vi "假的lumitrax.vi"() -> ()   [LabVIEW 2015]
uses:
  <vilib>/vision/NI_Vision_Development_Module.lvlib
panel:
  out "Image 2":T1(plugin-control)
  out "Image":T1(plugin-control)
  out "x-y":dbl
  out "Left":T1(plugin-control)
  out "Up":T1(plugin-control)
  out "Right":T1(plugin-control)
  out "Down":T1(plugin-control)
  out "Array":T1[][](array[plugin-control])
  out "UD":T1(plugin-control)
  out "Ave":T1(plugin-control)
  out "UDLR":T1(plugin-control)
  out "LR":T1(plugin-control)
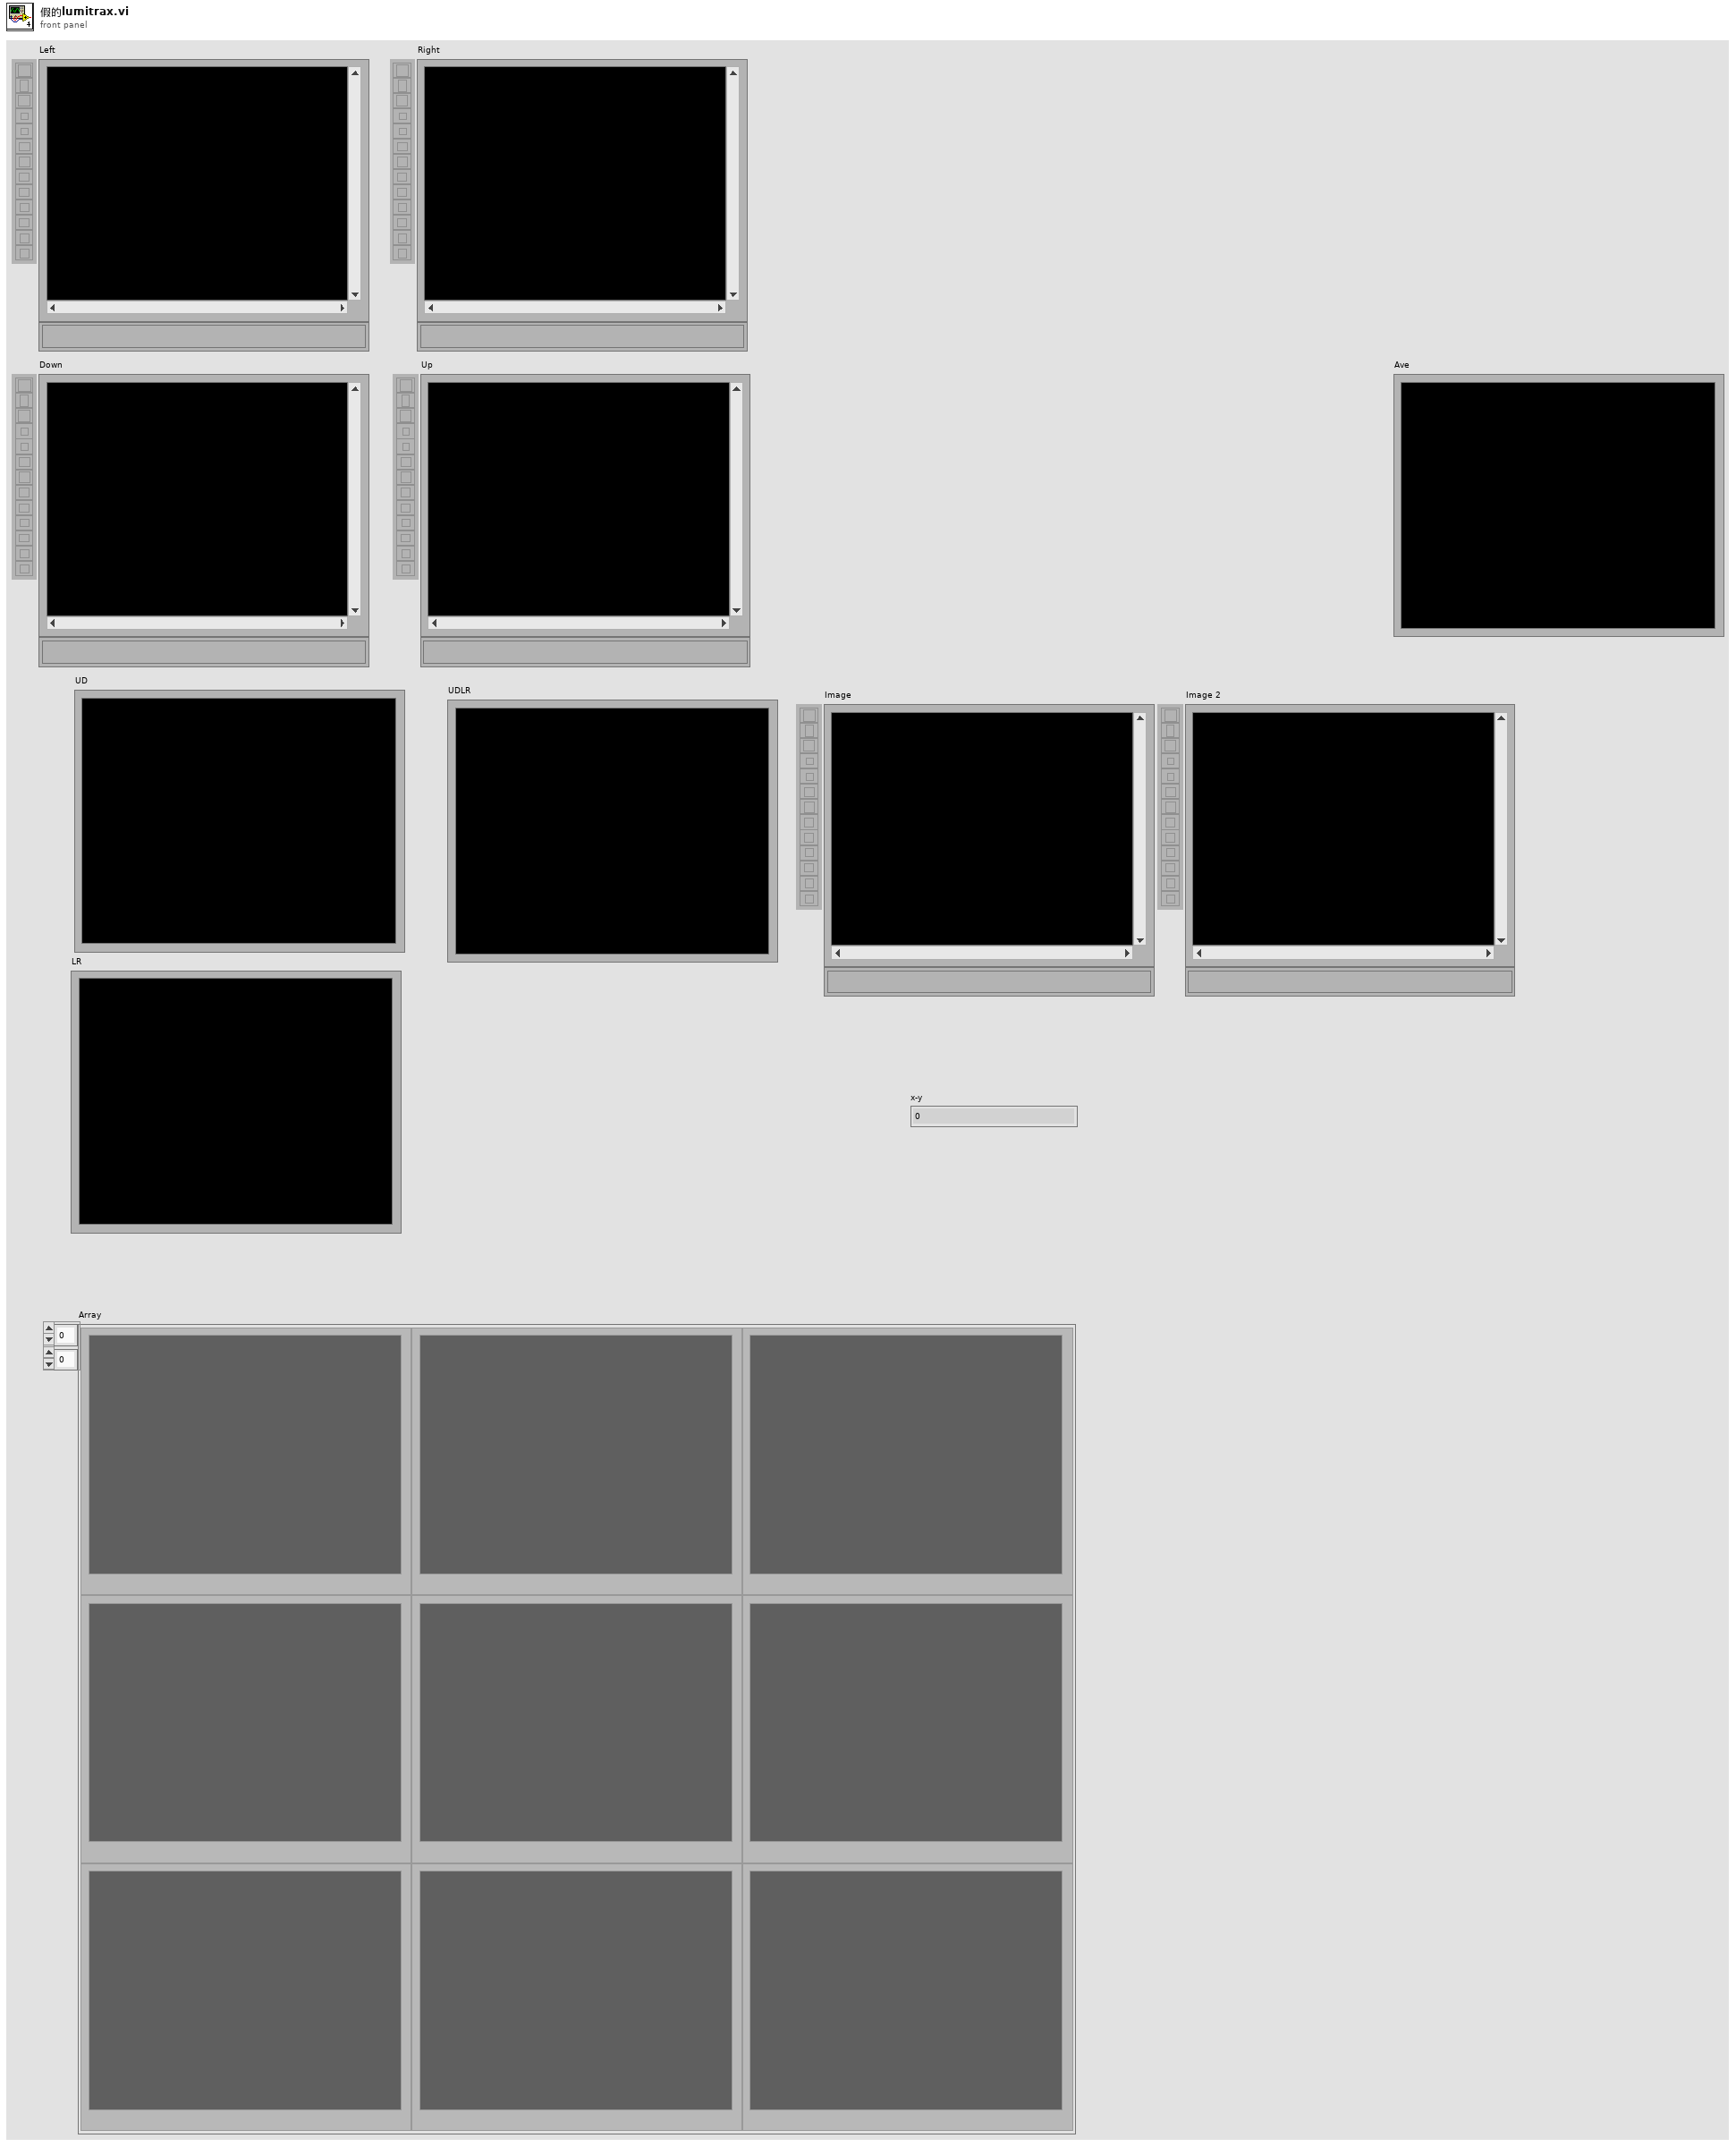
[diagram p1: front panel]
types:
  T1 = typedef "IMAQ Image.ctl" = refnum<image>
  T2 = cluster{"Line Scan Image?":bool, "Correction Factor":sgl}
  T3 = cluster{"Model":i32, "Sampling Grid Size":cluster{"SizeX":i32, "SizeY":i32}, "Polynomial Degree":i32}
  T4 = cluster{"Estimate Background?":bool, "Method":i32, "Polynomial Degree":i32, "Window Size (32x32)":cluster{"SizeX":i32, "SizeY":i32}, "Niblack Deviation Factor (0.2)":dbl}
  T5 = typedef "Image Type" = u32
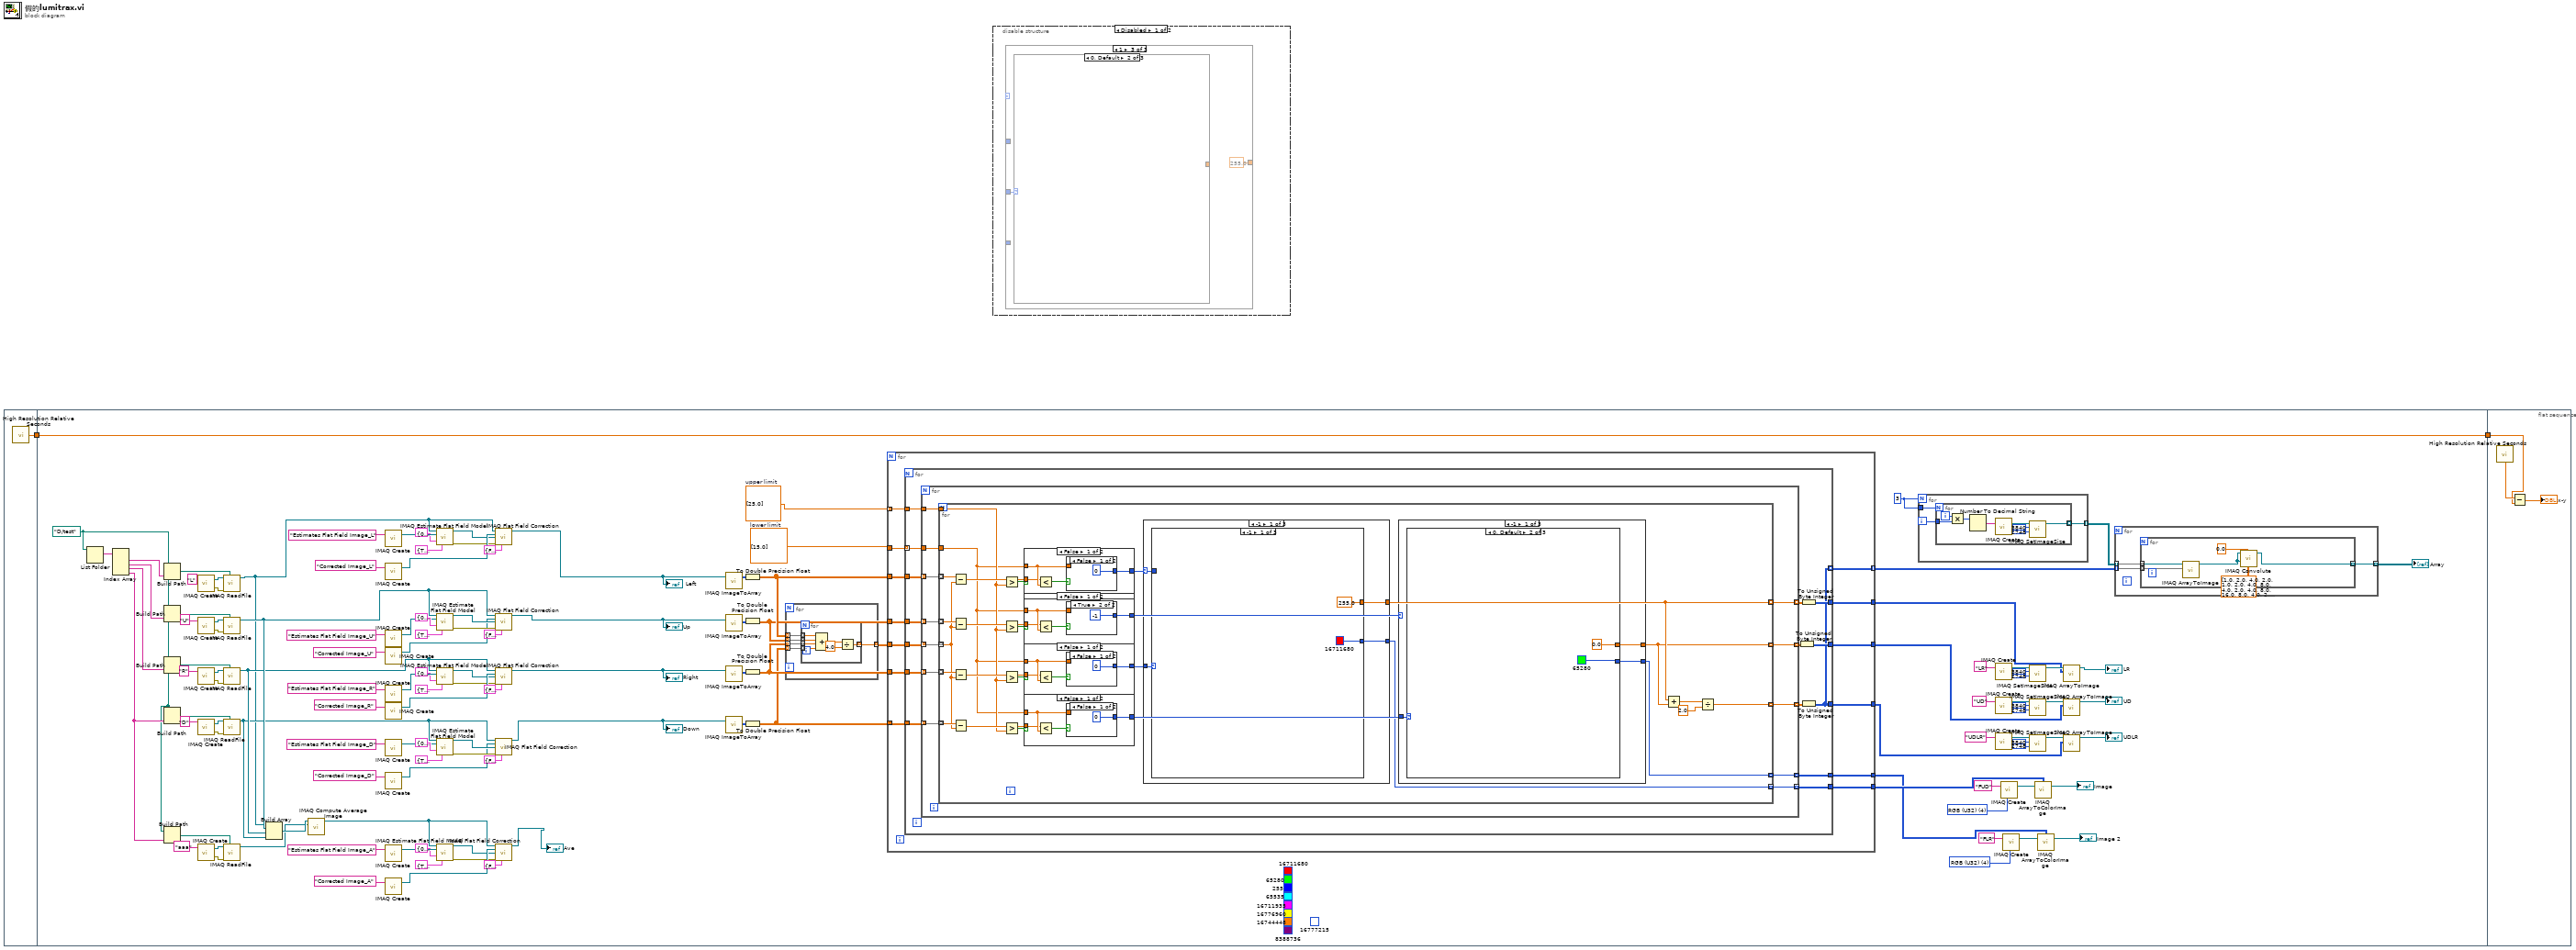
[diagram p0: block diagram]
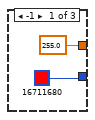
[diagram p2: hidden frame]
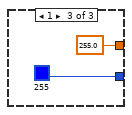
[diagram p3: hidden frame]
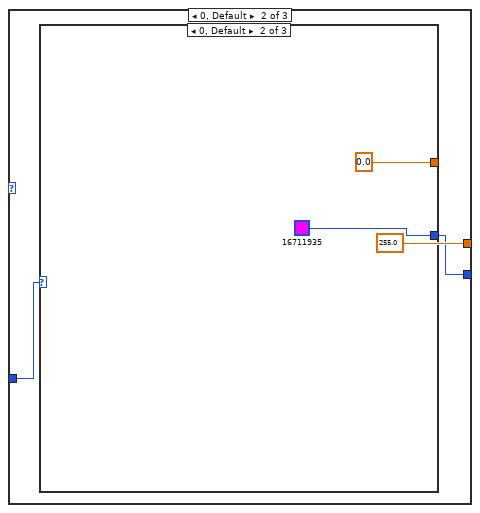
[diagram p4: hidden frame]
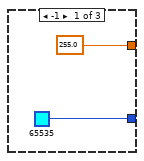
[diagram p5: hidden frame]
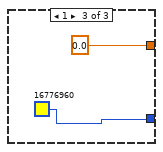
[diagram p6: hidden frame]
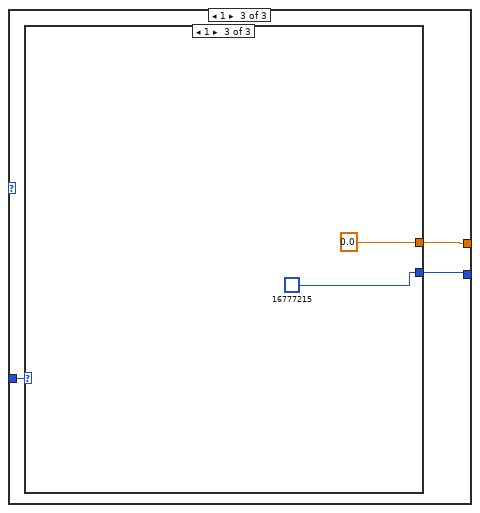
[diagram p7: hidden frame]
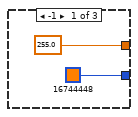
[diagram p8: hidden frame]
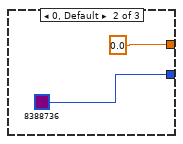
[diagram p9: hidden frame]
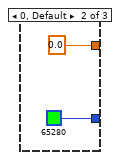
[diagram p10: hidden frame]
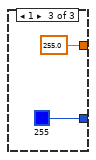
[diagram p11: hidden frame]
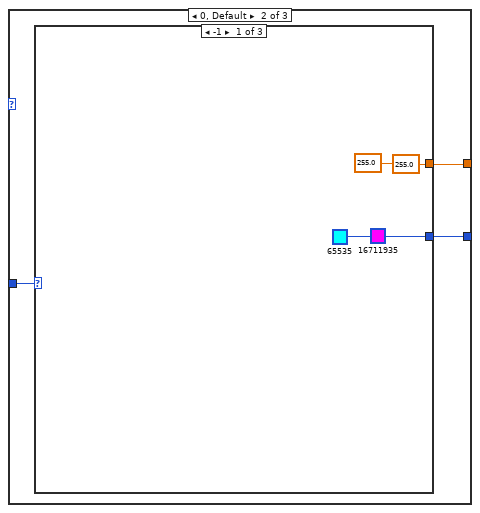
[diagram p12: hidden frame]
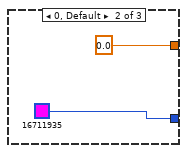
[diagram p13: hidden frame]
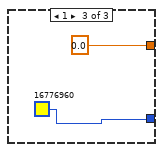
[diagram p14: hidden frame]
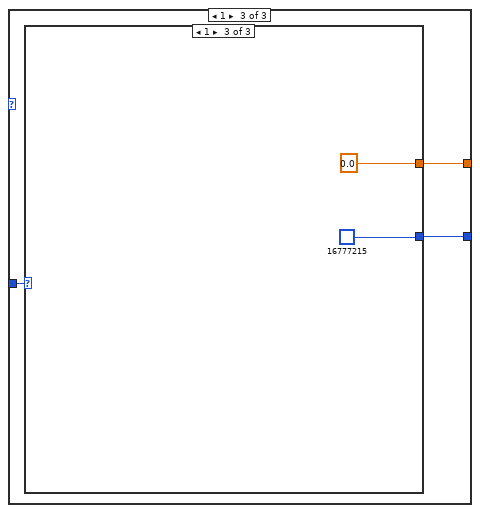
[diagram p15: hidden frame]
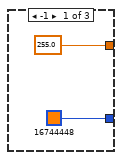
[diagram p16: hidden frame]
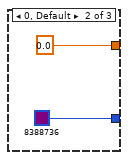
[diagram p17: hidden frame]
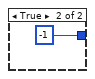
[diagram p18: hidden frame]
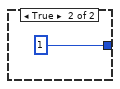
[diagram p19: hidden frame]
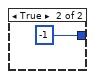
[diagram p20: hidden frame]
diagram:
  n1 = flat-sequence {
    tunnel: [w3] -> w2
    tunnel: w2 -> [w16]
    tunnel: [w16] -> w1
    tunnel: w1 -> [w316]
    frame #0 {
      n2 = call <vilib>:"High Resolution Relative Seconds.vi"() -> ("relative seconds"=w3:dbl)
    }
    frame #1 {
      w8 = T5 4 items=["Grayscale (U8)", "Grayscale (I16)", "Grayscale (SGL)", "Complex (CSG)", "RGB (U32)", "HSL (U32)", "RGB (U64)", "Grayscale (U16)"] ("Image Type")
      w9 = T5 4 items=["Grayscale (U8)", "Grayscale (I16)", "Grayscale (SGL)", "Complex (CSG)", "RGB (U32)", "HSL (U32)", "RGB (U64)", "Grayscale (U16)"] ("Image Type")
      (unwired) u32 16777215 ("O")
      (unwired) u32 8388736 ("P")
      (unwired) u32 16744448 ("O")
      (unwired) u32 16776960 ("Y")
      (unwired) u32 65535 ("C")
      (unwired) u32 16711935 ("M")
      (unwired) u32 255 ("B")
      (unwired) u32 65280 ("G")
      (unwired) u32 16711680 ("R")
      w14 = dbl[] [15.0]  # lower limit
      w15 = dbl[] [25.0]  # upper limit
      w26 = path "D:/test"
      w121 = 3
      n3 = List Folder(path=w26) -> (filenames=w119:string[])  [unwired: 3 in, 3 out]
      n4 = Index Array(array=w119) -> (element #1=w118:string, element #2=w116:string, element #3=w117:string, element #4=w43:string)  [unwired: 4 in]
      n5 = Build Path(base path=w26, name or relative path=w118) -> (appended path=w115:path)
      n6 = Build Path(base path=w26, name or relative path=w116) -> (appended path=w114:path)
      n7 = Build Path(base path=w26, name or relative path=w117) -> (appended path=w113:path)
      n8 = Build Path(base path=w26, name or relative path=w43) -> (appended path=w112:path)
      n9 = Build Path(base path=w26, name or relative path=w43) -> (appended path=w47:path)
      n10 = call "IMAQ Create"("Image Name"="L") -> ("New Image"=w128:T1, "error out"=w129:errorcluster)  [unwired: 4 in]
      n11 = call "IMAQ Create"("Image Name"="U") -> ("New Image"=w126:T1, "error out"=w127:errorcluster)  [unwired: 4 in]
      n12 = call "IMAQ Create"("Image Name"="R") -> ("New Image"=w124:T1, "error out"=w125:errorcluster)  [unwired: 4 in]
      n13 = call "IMAQ Create"("Image Name"="D") -> ("New Image"=w122:T1, "error out"=w123:errorcluster)  [unwired: 4 in]
      n14 = call "IMAQ Create"("Image Name"="aaa") -> ("New Image"=w46:T1, "error out"=w45:errorcluster)  [unwired: 4 in]
      n15 = call "IMAQ ReadFile"("File Path"=w115, "error in (no error)"=w129, "Image"=w128) -> ("Image Out"=w27:T1)  [unwired: 4 in, 4 out]
      n16 = call "IMAQ ReadFile"("File Path"=w114, "error in (no error)"=w127, "Image"=w126) -> ("Image Out"=w42:T1)  [unwired: 4 in, 4 out]
      n17 = call "IMAQ ReadFile"("File Path"=w113, "error in (no error)"=w125, "Image"=w124) -> ("Image Out"=w41:T1)  [unwired: 4 in, 4 out]
      n18 = call "IMAQ ReadFile"("File Path"=w112, "error in (no error)"=w123, "Image"=w122) -> ("Image Out"=w40:T1)  [unwired: 4 in, 4 out]
      n19 = call "IMAQ ReadFile"("File Path"=w47, "error in (no error)"=w45, "Image"=w46) -> ("Image Out"=w38:T1)  [unwired: 4 in, 4 out]
      n20 = Build Array(w27, w42, w41, w40) -> (w39:T1[])
      n21 = call "IMAQ Compute Average Image"("Image Dst"=w38, "Images"=w39) -> ("Image Dst Out"=w28:T1)  [unwired: 8 in, 1 out]
      n22 = call "IMAQ Create"("Image Name"="Estimates Flat Field Image_L") -> ("New Image"=w84:T1)  [unwired: 4 in, 1 out]
      n23 = call "IMAQ Create"("Image Name"="Corrected Image_L") -> ("New Image"=w85:T1)  [unwired: 4 in, 1 out]
      n24 = call "IMAQ Create"("Image Name"="Estimates Flat Field Image_U") -> ("New Image"=w73:T1)  [unwired: 4 in, 1 out]
      n25 = call "IMAQ Create"("Image Name"="Corrected Image_U") -> ("New Image"=w72:T1)  [unwired: 4 in, 1 out]
      n26 = call "IMAQ Create"("Image Name"="Estimates Flat Field Image_R") -> ("New Image"=w66:T1)  [unwired: 4 in, 1 out]
      n27 = call "IMAQ Create"("Image Name"="Corrected Image_R") -> ("New Image"=w67:T1)  [unwired: 4 in, 1 out]
      n28 = call "IMAQ Create"("Image Name"="Estimates Flat Field Image_D") -> ("New Image"=w55:T1)  [unwired: 4 in, 1 out]
      n29 = call "IMAQ Create"("Image Name"="Corrected Image_D") -> ("New Image"=w54:T1)  [unwired: 4 in, 1 out]
      n30 = call "IMAQ Create"("Image Name"="Estimates Flat Field Image_A") -> ("New Image"=w35:T1)  [unwired: 4 in, 1 out]
      n31 = call "IMAQ Create"("Image Name"="Corrected Image_A") -> ("New Image"=w36:T1)  [unwired: 4 in, 1 out]
      n32 = call "IMAQ Estimate Flat Field Model"("Image Src"=w27, "Image Dst"=w84, "Surface Fit Options"=T3 {"Model"=0, "Sampling Grid Size"={"SizeX"=100, "SizeY"=100}, "Polynomial Degree"=3}, "Background Estimation Options"=T4 {"Estimate Background?"=TRUE, "Method"=0, "Polynomial Degree"=2, "Window Size (32x32)"={"SizeX"=32, "SizeY"=32}, "Niblack Deviation Factor (0.2)"=0.2}) -> ("Flat Field Image Out"=w83:T1, "error out"=w81:errorcluster)  [unwired: 10 in]
      n33 = call "IMAQ Estimate Flat Field Model"("Image Src"=w42, "Image Dst"=w73, "Surface Fit Options"=T3 {"Model"=0, "Sampling Grid Size"={"SizeX"=100, "SizeY"=100}, "Polynomial Degree"=3}, "Background Estimation Options"=T4 {"Estimate Background?"=TRUE, "Method"=0, "Polynomial Degree"=2, "Window Size (32x32)"={"SizeX"=32, "SizeY"=32}, "Niblack Deviation Factor (0.2)"=0.2}) -> ("Flat Field Image Out"=w74:T1, "error out"=w76:errorcluster)  [unwired: 10 in]
      n34 = call "IMAQ Estimate Flat Field Model"("Image Src"=w41, "Image Dst"=w66, "Surface Fit Options"=T3 {"Model"=0, "Sampling Grid Size"={"SizeX"=100, "SizeY"=100}, "Polynomial Degree"=3}, "Background Estimation Options"=T4 {"Estimate Background?"=TRUE, "Method"=0, "Polynomial Degree"=2, "Window Size (32x32)"={"SizeX"=32, "SizeY"=32}, "Niblack Deviation Factor (0.2)"=0.2}) -> ("Flat Field Image Out"=w65:T1, "error out"=w63:errorcluster)  [unwired: 10 in]
      n35 = call "IMAQ Estimate Flat Field Model"("Image Src"=w40, "Image Dst"=w55, "Surface Fit Options"=T3 {"Model"=0, "Sampling Grid Size"={"SizeX"=100, "SizeY"=100}, "Polynomial Degree"=3}, "Background Estimation Options"=T4 {"Estimate Background?"=TRUE, "Method"=0, "Polynomial Degree"=2, "Window Size (32x32)"={"SizeX"=32, "SizeY"=32}, "Niblack Deviation Factor (0.2)"=0.2}) -> ("Flat Field Image Out"=w56:T1, "error out"=w58:errorcluster)  [unwired: 10 in]
      n36 = call "IMAQ Estimate Flat Field Model"("Image Src"=w28, "Image Dst"=w35, "Surface Fit Options"=T3 {"Model"=0, "Sampling Grid Size"={"SizeX"=100, "SizeY"=100}, "Polynomial Degree"=3}, "Background Estimation Options"=T4 {"Estimate Background?"=TRUE, "Method"=0, "Polynomial Degree"=2, "Window Size (32x32)"={"SizeX"=32, "SizeY"=32}, "Niblack Deviation Factor (0.2)"=0.2}) -> ("Flat Field Image Out"=w34:T1, "error out"=w32:errorcluster)  [unwired: 10 in]
      n37 = call "IMAQ Flat Field Correction"("Image Src"=w27, "Image Dst"=w85, "Flat Field Image"=w83, "error in (no error)"=w81, "Correction Options"=T2 {"Line Scan Image?"=FALSE, "Correction Factor"=1.1}) -> ("Corrected Image"=w48:T1)  [unwired: 8 in, 2 out]
      "Left" <- w48
      n38 = call "IMAQ Flat Field Correction"("Image Src"=w42, "Image Dst"=w72, "Flat Field Image"=w74, "error in (no error)"=w76, "Correction Options"=T2 {"Line Scan Image?"=FALSE, "Correction Factor"=1.1}) -> ("Corrected Image"=w49:T1)  [unwired: 8 in, 2 out]
      "Up" <- w49
      n39 = call "IMAQ Flat Field Correction"("Image Src"=w41, "Image Dst"=w67, "Flat Field Image"=w65, "error in (no error)"=w63, "Correction Options"=T2 {"Line Scan Image?"=FALSE, "Correction Factor"=1.1}) -> ("Corrected Image"=w50:T1)  [unwired: 8 in, 2 out]
      "Right" <- w50
      n40 = call "IMAQ Flat Field Correction"("Image Src"=w40, "Image Dst"=w54, "Flat Field Image"=w56, "error in (no error)"=w58, "Correction Options"=T2 {"Line Scan Image?"=FALSE, "Correction Factor"=1.1}) -> ("Corrected Image"=w51:T1)  [unwired: 8 in, 2 out]
      "Down" <- w51
      n41 = call "IMAQ Flat Field Correction"("Image Src"=w28, "Image Dst"=w36, "Flat Field Image"=w34, "error in (no error)"=w32, "Correction Options"=T2 {"Line Scan Image?"=FALSE, "Correction Factor"=1.1}) -> ("Corrected Image"=→"Ave":T1)  [unwired: 8 in, 2 out]
      n42 = call "IMAQ ImageToArray"("Image"=w48) -> ("Image Pixels (U8)"=w111:u8[][])  [unwired: 3 in, 4 out]
      n43 = call "IMAQ ImageToArray"("Image"=w49) -> ("Image Pixels (U8)"=w110:u8[][])  [unwired: 3 in, 4 out]
      n44 = call "IMAQ ImageToArray"("Image"=w50) -> ("Image Pixels (U8)"=w109:u8[][])  [unwired: 3 in, 4 out]
      n45 = call "IMAQ ImageToArray"("Image"=w51) -> ("Image Pixels (U8)"=w108:u8[][])  [unwired: 3 in, 4 out]
      n46 = To Double Precision Float(number=w111) -> (double precision float=w107:dbl[][])
      n47 = To Double Precision Float(number=w110) -> (double precision float=w106:dbl[][])
      n48 = To Double Precision Float(number=w109) -> (double precision float=w105:dbl[][])
      n49 = To Double Precision Float(number=w108) -> (double precision float=w104:dbl[][])
      n50 = for {
        tunnel: w107 -> [w138] mode=indexing
        tunnel: w106 -> [w137] mode=indexing
        tunnel: w105 -> [w136] mode=indexing
        tunnel: w104 -> [w135] mode=indexing
        tunnel: [w134] -> w103 mode=indexing
        n51 = for {
          tunnel: w138 -> [w144] mode=indexing
          tunnel: w137 -> [w143] mode=indexing
          tunnel: w136 -> [w142] mode=indexing
          tunnel: w135 -> [w141] mode=indexing
          tunnel: [w140] -> w134 mode=indexing
          n52 = Compound Arithmetic op=ADD(w144, w143, w142, w141) -> (w145:dbl)
          n53 = Divide(x=w145, y=4.0) -> (x/y=w140:dbl)
        }
      }
      n54 = for {
        tunnel: w107 -> [w178]
        tunnel: w106 -> [w177]
        tunnel: w105 -> [w176]
        tunnel: w104 -> [w175]
        tunnel: w15 -> [w174] mode=indexing
        tunnel: w14 -> [w173]
        tunnel: w103 -> [w172]
        tunnel: [w171] -> w101 mode=indexing
        tunnel: [w170] -> w89
        tunnel: [w169] -> w90
        tunnel: [w168] -> w20
        tunnel: [w167] -> w10
        tunnel: [w166] -> w4
        n55 = for {
          tunnel: w178 -> [w192]
          tunnel: w177 -> [w191]
          tunnel: w176 -> [w190]
          tunnel: w175 -> [w189]
          tunnel: w174 -> [w188]
          tunnel: w173 -> [w187] mode=indexing
          tunnel: [w186] -> w169
          tunnel: w172 -> [w185]
          tunnel: [w181] -> w171 mode=indexing
          tunnel: [w183] -> w170
          tunnel: [w181] -> w168
          tunnel: [w180] -> w167
          tunnel: [w179] -> w166
          n56 = for {
            tunnel: w192 -> [w205] mode=indexing
            tunnel: w191 -> [w204] mode=indexing
            tunnel: w190 -> [w203] mode=indexing
            tunnel: w189 -> [w202] mode=indexing
            tunnel: [w201] -> w193 mode=indexing
            tunnel: w188 -> [w200]
            tunnel: w187 -> [w199]
            tunnel: w185 -> [w198] mode=indexing
            tunnel: [w197] -> w184 mode=indexing
            tunnel: [w196] -> w182 mode=indexing
            tunnel: [w195] -> w180 mode=indexing
            tunnel: [w194] -> w179 mode=indexing
            n57 = for {
              tunnel: w205 -> [w231] mode=indexing
              tunnel: w204 -> [w230] mode=indexing
              tunnel: w203 -> [w229] mode=indexing
              tunnel: w202 -> [w228] mode=indexing
              tunnel: [w208] -> w201 mode=indexing
              tunnel: w200 -> [w217]
              tunnel: w199 -> [w216]
              tunnel: w198 -> [w215] mode=indexing
              tunnel: [w210] -> w197 mode=indexing
              tunnel: [w209] -> w196 mode=indexing
              tunnel: [w207] -> w195 mode=indexing
              tunnel: [w206] -> w194 mode=indexing
              n58 = Subtract(x=w231, y=w215) -> (x-y=w223:dbl)
              n59 = Subtract(x=w230, y=w215) -> (x-y=w219:dbl)
              n60 = Subtract(x=w229, y=w215) -> (x-y=w218:dbl)
              n61 = Subtract(x=w228, y=w215) -> (x-y=w222:dbl)
              n62 = Greater?(x=w223, y=w217) -> (0:w227:bool)
              n63 = Greater?(x=w219, y=w217) -> (0:w226:bool)
              n64 = Greater?(x=w218, y=w217) -> (0:w225:bool)
              n65 = Greater?(x=w222, y=w217) -> (0:w224:bool)
              n66 = case shown="False" w227 {
                tunnel: w216 -> [w311 _]
                tunnel: w223 -> [w310 _]
                tunnel: [w308 1] -> w221
                frame False {
                  n67 = Less?(x=w310, y=w311) -> (x < y?=w309:bool)
                  n68 = case shown="False" w309 {
                    tunnel: w311 -> [_ _]
                    tunnel: [0 -1] -> w308
                    frame False {
                    }
                    frame True {
                    }
                  }
                }
                frame True {
                }
              }
              n69 = case shown="False" w226 {
                tunnel: w216 -> [w304 _]
                tunnel: w219 -> [w303 _]
                tunnel: [w301 1] -> w214
                frame False {
                  n70 = Less?(x=w303, y=w304) -> (x < y?=w302:bool)
                  n71 = case shown="True" w302 {
                    tunnel: w304 -> [_ _]
                    tunnel: [0 -1] -> w301
                    frame False {
                    }
                    frame True {
                    }
                  }
                }
                frame True {
                }
              }
              n72 = case shown="False" w225 {
                tunnel: w216 -> [w297 _]
                tunnel: w218 -> [w296 _]
                tunnel: [w294 1] -> w220
                frame False {
                  n73 = Less?(x=w296, y=w297) -> (x < y?=w295:bool)
                  n74 = case shown="False" w295 {
                    tunnel: w297 -> [_ _]
                    tunnel: [0 -1] -> w294
                    frame False {
                    }
                    frame True {
                    }
                  }
                }
                frame True {
                }
              }
              n75 = case shown="False" w224 {
                tunnel: w216 -> [w290 _]
                tunnel: w222 -> [w289 _]
                tunnel: [w287 1] -> w213
                frame False {
                  n76 = Less?(x=w289, y=w290) -> (x < y?=w288:bool)
                  n77 = case shown="False" w288 {
                    tunnel: w290 -> [_ _]
                    tunnel: [0 -1] -> w287
                    frame False {
                    }
                    frame True {
                    }
                  }
                }
                frame True {
                }
              }
              n78 = case shown="-1" w221 {
                selector: w221 -> [w261 _ _]
                tunnel: w220 -> [w262 w270 w280]
                tunnel: [w260 255.0 w279] -> w210
                tunnel: [w259 w269 w278] -> w207
                frame -1 {
                  n79 = case shown="-1" w262 {
                    tunnel: [255.0 0.0 255.0] -> w260
                    tunnel: w261 -> [_ _ _]
                    tunnel: [u32 16711680 ("R") u32 65280 ("G") u32 255 ("B")] -> w259
                    frame -1 {
                    }
                    frame 0, Default {
                    }
                    frame 1 {
                    }
                  }
                }
                frame 0, Default {
                  (unwired) u32 16711935 ("M")
                  n80 = case shown="-1" w270 {
                    tunnel: [255.0 0.0 0.0] -> _
                    tunnel: [u32 65535 ("C") u32 16711935 ("M") u32 16776960 ("Y")] -> w269
                    frame -1 {
                    }
                    frame 0, Default {
                    }
                    frame 1 {
                    }
                  }
                }
                frame 1 {
                  n81 = case shown="1" w280 {
                    tunnel: [255.0 0.0 0.0] -> w279
                    tunnel: [u32 16744448 ("O") u32 8388736 ("P") u32 16777215 ("O")] -> w278
                    frame -1 {
                    }
                    frame 0, Default {
                    }
                    frame 1 {
                    }
                  }
                }
              }
              n82 = case shown="-1" w214 {
                tunnel: w213 -> [w233 w241 w252]
                tunnel: [w234 255.0 w251] -> w208
                tunnel: [w232 w242 w250] -> w206
                frame -1 {
                  n83 = case shown="0, Default" w233 {
                    tunnel: [255.0 0.0 255.0] -> w234
                    tunnel: [u32 16711680 ("B") u32 65280 ("R") u32 255 ("G")] -> w232
                    frame -1 {
                    }
                    frame 0, Default {
                    }
                    frame 1 {
                    }
                  }
                }
                frame 0, Default {
                  n84 = case shown="0, Default" w241 {
                    tunnel: [255.0 0.0 0.0] -> _
                    tunnel: [u32 65535 ("C") u32 16711935 ("M") u32 16776960 ("Y")] -> w242
                    frame -1 {
                    }
                    frame 0, Default {
                    }
                    frame 1 {
                    }
                  }
                }
                frame 1 {
                  n85 = case shown="1" w252 {
                    tunnel: [255.0 0.0 0.0] -> w251
                    tunnel: [u32 16744448 ("O") u32 8388736 ("P") u32 16777215 ("O")] -> w250
                    frame -1 {
                    }
                    frame 0, Default {
                    }
                    frame 1 {
                    }
                  }
                }
              }
              n86 = Add(x=w210, y=w208) -> (x+y=w212:dbl)
              n87 = Divide(x=w212, y=2.0) -> (x/y=w209:dbl)
            }
          }
          n88 = To Unsigned Byte Integer(number=w193) -> (unsigned 8bit integer=w186:u8[][])
          n89 = To Unsigned Byte Integer(number=w184) -> (unsigned 8bit integer=w183:u8[][])
          n90 = To Unsigned Byte Integer(number=w182) -> (unsigned 8bit integer=w181:u8[][])
        }
      }
      n91 = for {
        N: w121 -> [_]
        tunnel: w121 -> [w148]
        tunnel: [w146] -> w102 mode=indexing
        i -> [w147]
        n92 = for {
          N: w148 -> [_]
          tunnel: w147 -> [w152]
          tunnel: [w149] -> w146 mode=indexing
          i -> [w153]
          n93 = Multiply(x=w153, y=w152) -> (x*y=w151:i32)
          n94 = Number To Decimal String(number=w151) -> (decimal integer string=w150:string)  [unwired: 1 in]
          n95 = call "IMAQ Create"("Image Name"=w150) -> ("New Image"=w155:T1)  [unwired: 4 in, 1 out]
          n96 = call "IMAQ SetImageSize"("Y Resolution"=2748 ("X Resolution"), "X Resolution"=3840, "Image"=w155) -> ("Image Out"=w149:T1)  [unwired: 2 in, 1 out]
        }
      }
      n97 = call "IMAQ Create"("Image Name"="LR") -> ("New Image"=w99:T1)  [unwired: 4 in, 1 out]
      n98 = call "IMAQ Create"("Image Name"="UD") -> ("New Image"=w96:T1)  [unwired: 4 in, 1 out]
      n99 = call "IMAQ Create"("Image Name"="UDLR") -> ("New Image"=w22:T1)  [unwired: 4 in, 1 out]
      n100 = call "IMAQ Create"("Image Name"="FUD", "Image Type"=w9) -> ("New Image"=w11:T1)  [unwired: 3 in, 1 out]
      n101 = call "IMAQ Create"("Image Name"="FLR", "Image Type"=w8) -> ("New Image"=w7:T1)  [unwired: 3 in, 1 out]
      n102 = call "IMAQ SetImageSize"("Y Resolution"=2748 ("X Resolution"), "X Resolution"=3840, "Image"=w99) -> ("Image Out"=w92:T1)  [unwired: 2 in, 1 out]
      n103 = call "IMAQ SetImageSize"("Y Resolution"=2748 ("X Resolution"), "X Resolution"=3840, "Image"=w96) -> ("Image Out"=w91:T1)  [unwired: 2 in, 1 out]
      n104 = call "IMAQ SetImageSize"("Y Resolution"=2748 ("X Resolution"), "X Resolution"=3840, "Image"=w22) -> ("Image Out"=w25:T1)  [unwired: 2 in, 1 out]
      n105 = call "IMAQ ArrayToColorImage"("Image Pixels (U32)"=w10, "Image"=w11) -> ("Image Out"=→"Image":T1)  [unwired: 3 in, 1 out]
      n106 = call "IMAQ ArrayToColorImage"("Image Pixels (U32)"=w4, "Image"=w7) -> ("Image Out"=→"Image 2":T1)  [unwired: 3 in, 1 out]
      n107 = call "IMAQ ArrayToImage"("Image Pixels (U8)"=w89, "Image"=w92) -> ("Image Out"=→"LR":T1)  [unwired: 8 in, 1 out]
      n108 = call "IMAQ ArrayToImage"("Image Pixels (U8)"=w90, "Image"=w91) -> ("Image Out"=→"UD":T1)  [unwired: 8 in, 1 out]
      n109 = call "IMAQ ArrayToImage"("Image Pixels (U8)"=w20, "Image"=w25) -> ("Image Out"=→"UDLR":T1)  [unwired: 8 in, 1 out]
      n110 = for {
        tunnel: w101 -> [w159] mode=indexing
        tunnel: w102 -> [w158] mode=indexing
        tunnel: [w157] -> w120 mode=indexing
        n111 = for {
          tunnel: w159 -> [w164] mode=indexing
          tunnel: w158 -> [w165] mode=indexing
          tunnel: [w161] -> w157 mode=indexing
          n112 = call "IMAQ ArrayToImage"("Image Pixels (U8)"=w164, "Image"=w165) -> ("Image Out"=w160:T1)  [unwired: 8 in, 1 out]
          n113 = call "IMAQ Convolute"("Kernel"=sgl[][] [[1.0, 2.0, 4.0, 2.0, 1.0], [2.0, 4.0, 8.0, 4.0, 2.0], [4.0, 8.0, 16.0, 8.0, 4.0], [2.0, 4.0, 8.0, 4.0, 2.0], [1.0, 2.0, 4.0, 2.0, 1.0]], "Divider (kernel sum)"=sgl 0.0 ("Divider"), "Image Dst"=w160, "Image Src"=w160) -> ("Image Dst Out"=w161:T1)  [unwired: 3 in, 4 out]
        }
      }
      "Array" <- w120
    }
    frame #2 {
      n114 = call <vilib>:"High Resolution Relative Seconds.vi"() -> ("relative seconds"=w317:dbl)
      n115 = Subtract(x=w317, y=w316) -> (x-y=→"x-y":dbl)
    }
  }
  n116 = disable-structure shown="Disabled" {
    frame Disabled {
      n117 = case shown="1" {
        selector: _ -> [_ _ _]
        tunnel: _ -> [_ w322 _]
        tunnel: _ -> [_ w321 w335]
        tunnel: _ -> [_ w320 _]
        tunnel: [0.0 w319 255.0] -> _
        frame -1 {
        }
        frame 0, Default {
          n118 = case shown="0, Default" w322 {
            tunnel: w321 -> [_ w326 _]
            tunnel: w320 -> [_ w325 _]
            tunnel: [32.0 w324 255.0] -> w319
            frame -1 {
            }
            frame 0, Default {
              n119 = case shown="0, Default" w326 {
                tunnel: w325 -> [_ w329 _]
                tunnel: [64.0 w328 255.0] -> w324
                frame -1 {
                }
                frame 0, Default {
                  n120 = case shown="1" w329 {
                    tunnel: [128.0 192.0 255.0] -> w328
                    frame -1 {
                    }
                    frame 0, Default {
                    }
                    frame 1 {
                    }
                  }
                }
                frame 1 {
                }
              }
            }
            frame 1 {
            }
          }
        }
        frame 1 {
          n121 = case shown="0, Default" w335 {
            tunnel: [32.0 _ 255.0] -> _
            frame -1 {
            }
            frame 0, Default {
            }
            frame 1 {
            }
          }
        }
      }
    }
    frame Enabled {
    }
  }
